vi "Append To Dataset 3D Double.vi"(8 "Error in (no error)":errorcluster, 10 "Data":dbl[][][](array[numeric]), 11 "Dataset id in":i32) -> (0 "Error out":errorcluster, 3 "Dataset id out":i32)   [LabVIEW 2014]
uses:
  Release/HDF5Tools.dll
  HDF5Tools.lvlib
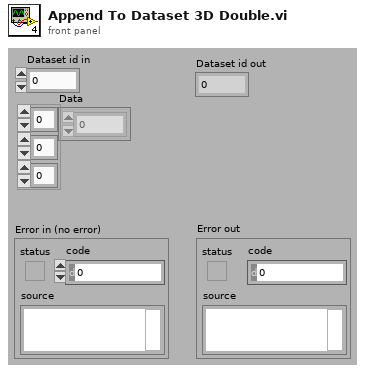
[diagram p1: front panel]
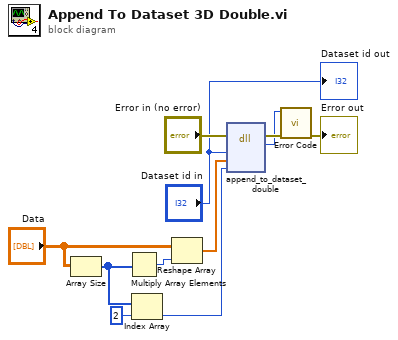
[diagram p0: block diagram]
diagram:
  n1 = Array Size(array="Data") -> (size(s)=w5:i32[])
  n2 = Multiply Array Elements(1:w5) -> (0:w3:i32)
  n3 = Index Array(array=w5, index=2) -> (element=w1:i32)
  n4 = Reshape Array("Data", w3) -> (w10:dbl[])
  n5 = dll-call lib="Z:/users/Manolis/Labview/Cajal/private/HDF5Tools32/Release/HDF5Tools.dll" fn="append_to_dataset_double"(error in="Error in (no error)", "dataset_id"="Dataset id in", "data"=w10, "count"=w1) -> (error out=w8:errorcluster, "error"=w7:i32)  [unwired: 5 in, 1 out]
  n6 = call "Error Code.vi"("Error in"=w8, "Error code"=w7) -> ("Error out"=→"Error out":errorcluster)  [unwired: 9 in]
  "Dataset id out" <- "Dataset id in"
